vi "Initial Picture.vi"(10 "中心位置":T1={"Cent X"=273.0, "Cent Y"=255.0, "Big1 R"=250.0, "Small1 R"=180.0, "Big2 R"=170.0, "Small2 R"=100.0, "Start_OutSide"=0.1, "Start_InSide"=0.1} {"Start_InSide" min=0.1 max=180.0; "Start_OutSide" min=0.1 max=180.0}, 11 "Image In":T2(plugin-control)) -> (0 "Outside Precent":string, 1 "Inside Precent":string, 3 "Image Out":T2(plugin-control))   [LabVIEW 2015]
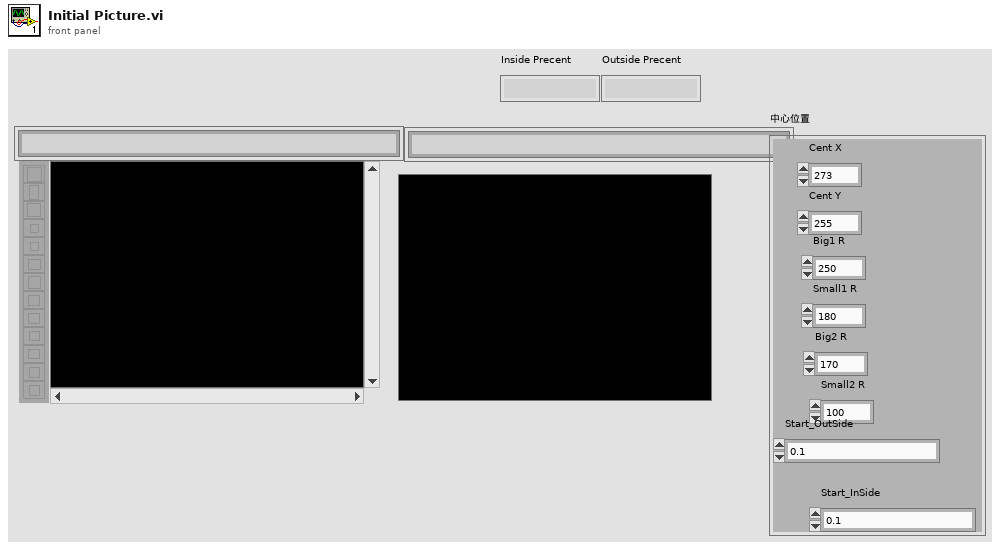
[diagram p1: front panel]
types:
  T1 = cluster{"Cent X":dbl, "Cent Y":dbl, "Big1 R":dbl, "Small1 R":dbl, "Big2 R":dbl, "Small2 R":dbl, "Start_OutSide":dbl, "Start_InSide":dbl}
  T2 = typedef "IMAQ Image.ctl" = refnum<image>
  T3 = cluster{"Left":i32, "Top":i32, "Right":i32, "Bottom":i32}
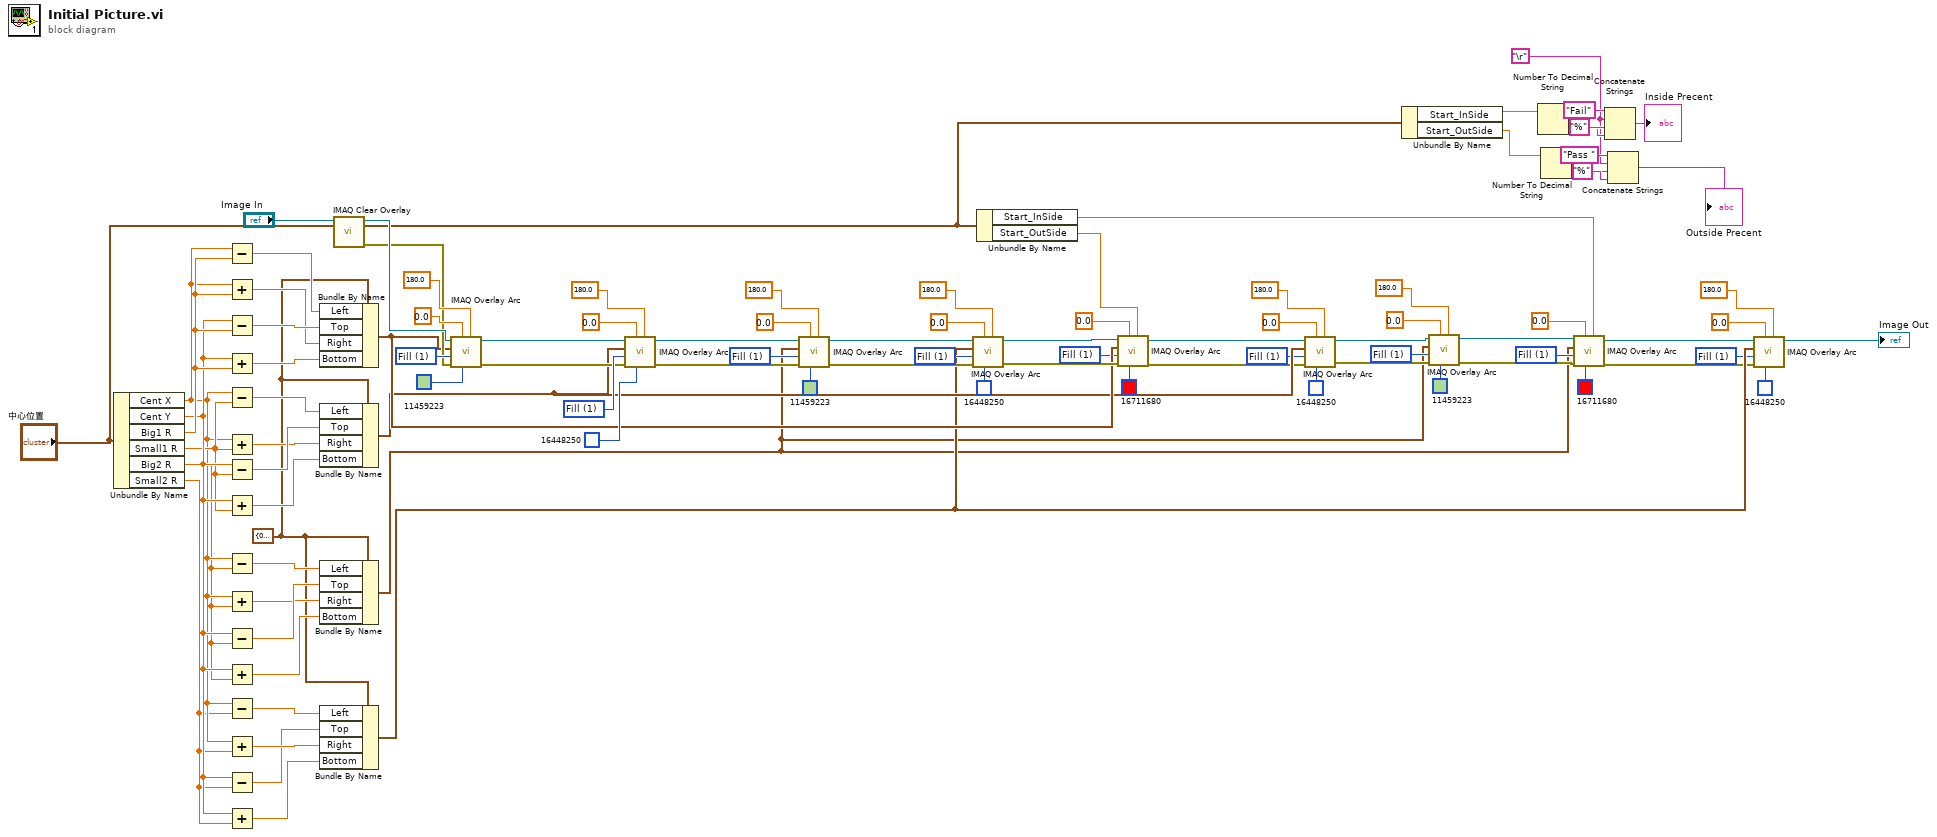
[diagram p0: block diagram]
diagram:
  w1 = "\r"
  w22 = u32 1 items=["Frame", "Fill"] ("Drawing Mode (Frame)")
  w29 = u32 1 items=["Frame", "Fill"] ("Drawing Mode (Frame)")
  w25 = u32 1 items=["Frame", "Fill"] ("Drawing Mode (Frame)")
  w36 = u32 1 items=["Frame", "Fill"] ("Drawing Mode (Frame)")
  w40 = u32 1 items=["Frame", "Fill"] ("Drawing Mode (Frame)")
  w67 = u32 1 items=["Frame", "Fill"] ("Drawing Mode (Frame)")
  w73 = u32 1 items=["Frame", "Fill"] ("Drawing Mode (Frame)")
  w49 = T3 {"Left"=0, "Top"=0, "Right"=0, "Bottom"=0} ("Bounding Rectangle")
  w90 = u32 1 items=["Frame", "Fill"] ("Drawing Mode (Frame)")
  w93 = u32 1 items=["Frame", "Fill"] ("Drawing Mode (Frame)")
  n1 = Unbundle By Name("中心位置") -> ("Cent X"=w52:dbl, "Cent Y"=w54:dbl, "Big1 R"=w75:dbl, "Small1 R"=w53:dbl, "Big2 R"=w51:dbl, "Small2 R"=w50:dbl)
  n2 = Subtract(x=w52, y=w75) -> (x-y=w83:dbl)
  n3 = Add(x=w52, y=w75) -> (x+y=w81:dbl)
  n4 = Subtract(x=w54, y=w75) -> (x-y=w82:dbl)
  n5 = Add(x=w54, y=w75) -> (x+y=w80:dbl)
  n6 = Subtract(x=w52, y=w53) -> (x-y=w79:dbl)
  n7 = Add(x=w52, y=w53) -> (x+y=w77:dbl)
  n8 = Subtract(x=w54, y=w53) -> (x-y=w78:dbl)
  n9 = Add(x=w54, y=w53) -> (x+y=w76:dbl)
  n10 = Subtract(x=w52, y=w51) -> (x-y=w62:dbl)
  n11 = Add(x=w52, y=w51) -> (x+y=w60:dbl)
  n12 = Subtract(x=w54, y=w51) -> (x-y=w61:dbl)
  n13 = Add(x=w54, y=w51) -> (x+y=w59:dbl)
  n14 = Subtract(x=w52, y=w50) -> (x-y=w55:dbl)
  n15 = Add(x=w52, y=w50) -> (x+y=w57:dbl)
  n16 = Subtract(x=w54, y=w50) -> (x-y=w56:dbl)
  n17 = Add(x=w54, y=w50) -> (x+y=w58:dbl)
  n18 = Bundle By Name(cluster=w49, "Left"=w83, "Top"=w82, "Right"=w81, "Bottom"=w80) -> (w44:T3)
  n19 = Bundle By Name(cluster=w49, "Left"=w79, "Top"=w78, "Right"=w77, "Bottom"=w76) -> (w43:T3)
  n20 = Bundle By Name(cluster=w49, "Left"=w62, "Top"=w61, "Right"=w60, "Bottom"=w59) -> (w15:T3)
  n21 = Bundle By Name(cluster=w49, "Left"=w55, "Top"=w56, "Right"=w57, "Bottom"=w58) -> (w42:T3)
  n22 = call "IMAQ Clear Overlay"("Image"="Image In") -> ("error out"=w48:errorcluster, "Image Out"=w84:T2)  [unwired: 9 in]
  n23 = call "IMAQ Overlay Arc"("End Angle (degrees)"=180.0, "Color"=u32 11459223, "Start Angle (degrees)"=0.0, "error in (no error)"=w48, "Drawing Mode (Frame)"=w93, "Bounding Rectangle"=w44, "Image"=w84) -> ("error out"=w86:errorcluster, "Image Out"=w87:T2)  [unwired: 3 in]
  n24 = call "IMAQ Overlay Arc"("End Angle (degrees)"=180.0, "Color"=u32 16448250, "Start Angle (degrees)"=0.0, "error in (no error)"=w86, "Drawing Mode (Frame)"=w90, "Bounding Rectangle"=w43, "Image"=w87) -> ("error out"=w63:errorcluster, "Image Out"=w70:T2)  [unwired: 3 in]
  n25 = call "IMAQ Overlay Arc"("End Angle (degrees)"=180.0, "Color"=u32 11459223, "Start Angle (degrees)"=0.0, "error in (no error)"=w63, "Drawing Mode (Frame)"=w73, "Bounding Rectangle"=w15, "Image"=w70) -> ("error out"=w64:errorcluster, "Image Out"=w65:T2)  [unwired: 3 in]
  n26 = call "IMAQ Overlay Arc"("End Angle (degrees)"=180.0, "Color"=u32 16448250, "Start Angle (degrees)"=0.0, "error in (no error)"=w64, "Drawing Mode (Frame)"=w67, "Bounding Rectangle"=w42, "Image"=w65) -> ("error out"=w46:errorcluster, "Image Out"=w47:T2)  [unwired: 3 in]
  n27 = Unbundle By Name("中心位置") -> ("Start_InSide"=w13:dbl, "Start_OutSide"=w14:dbl)
  n28 = call "IMAQ Overlay Arc"("End Angle (degrees)"=w14, "Color"=u32 16711680, "Start Angle (degrees)"=0.0, "error in (no error)"=w46, "Drawing Mode (Frame)"=w40, "Bounding Rectangle"=w44, "Image"=w47) -> ("error out"=w33:errorcluster, "Image Out"=w34:T2)  [unwired: 3 in]
  n29 = call "IMAQ Overlay Arc"("End Angle (degrees)"=180.0, "Color"=u32 16448250, "Start Angle (degrees)"=0.0, "error in (no error)"=w33, "Drawing Mode (Frame)"=w36, "Bounding Rectangle"=w43, "Image"=w34) -> ("error out"=w18:errorcluster, "Image Out"=w19:T2)  [unwired: 3 in]
  n30 = Unbundle By Name("中心位置") -> ("Start_InSide"=w12:dbl, "Start_OutSide"=w7:dbl)
  n31 = call "IMAQ Overlay Arc"("End Angle (degrees)"=180.0, "Color"=u32 11459223, "Start Angle (degrees)"=0.0, "error in (no error)"=w18, "Drawing Mode (Frame)"=w22, "Bounding Rectangle"=w15, "Image"=w19) -> ("error out"=w17:errorcluster, "Image Out"=w16:T2)  [unwired: 3 in]
  n32 = Number To Decimal String(number=w12) -> (decimal integer string=w11:string)  [unwired: 1 in]
  n33 = Number To Decimal String(number=w7) -> (decimal integer string=w8:string)  [unwired: 1 in]
  n34 = call "IMAQ Overlay Arc"("End Angle (degrees)"=w13, "Color"=u32 16711680, "Start Angle (degrees)"=0.0, "error in (no error)"=w17, "Drawing Mode (Frame)"=w25, "Bounding Rectangle"=w15, "Image"=w16) -> ("error out"=w32:errorcluster, "Image Out"=w31:T2)  [unwired: 3 in]
  n35 = Concatenate Strings("Fail" ("字符串"), w1, w11, "%" ("字符串")) -> (→"Inside Precent":string)
  n36 = Concatenate Strings("Pass " ("字符串"), w1, w8, "%" ("字符串")) -> (→"Outside Precent":string)
  n37 = call "IMAQ Overlay Arc"("End Angle (degrees)"=180.0, "Color"=u32 16448250, "Start Angle (degrees)"=0.0, "error in (no error)"=w32, "Drawing Mode (Frame)"=w29, "Bounding Rectangle"=w42, "Image"=w31) -> ("Image Out"=→"Image Out":T2)  [unwired: 3 in, 1 out]
